vi "ExcelImport.vi"(8 "错误输入（无错误）":errorcluster, 10 "Sheets":enum16{"Sheet1", "Sheet2", "Sheet3", "Sheet4"}(ring), 11 "路径":path) -> (0 "错误输出":errorcluster, 1 "After First":string[][](array[string]), 2 "First Row":string[](array[string]), 3 "All":string[][](array[string]))   [LabVIEW 2020]
panel:
  out "x-y":u32
  in  "Excel._Worksheet":refnum<k7>
  in  "Excel._Application":refnum<k7>
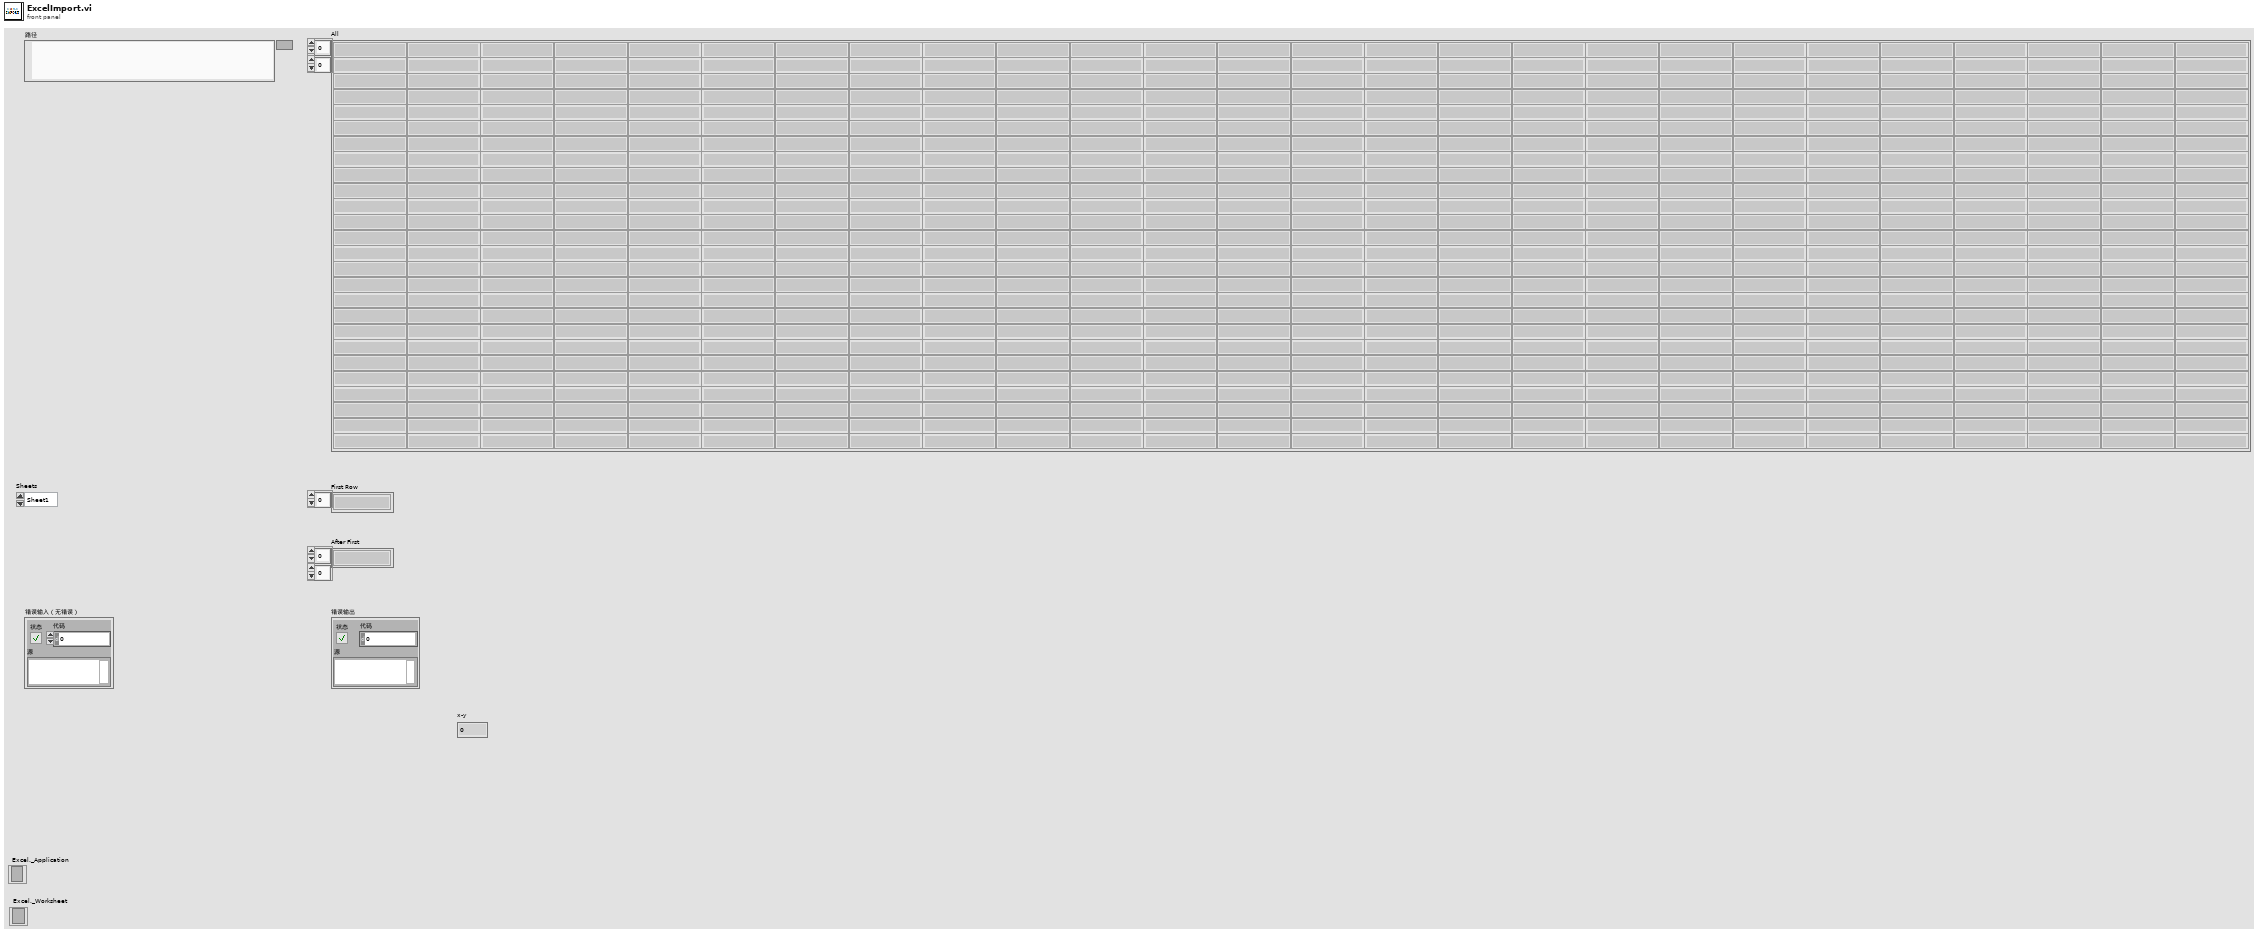
[diagram p1: front panel]
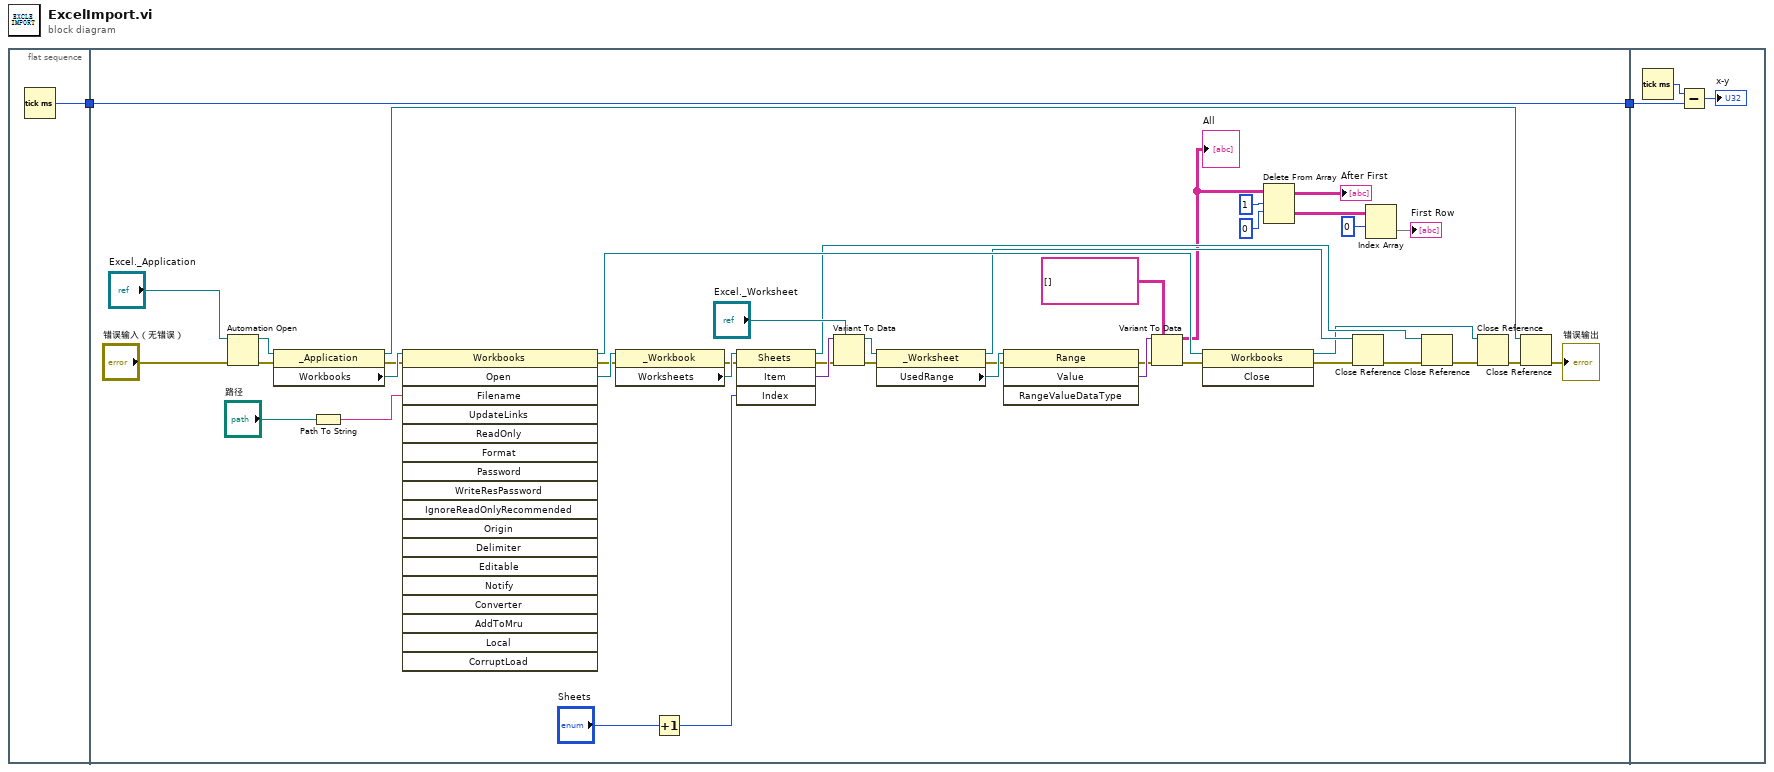
[diagram p0: block diagram]
diagram:
  n1 = flat-sequence {
    tunnel: [w3] -> w2
    tunnel: w2 -> [w10]
    tunnel: [w10] -> w1
    tunnel: w1 -> [w48]
    frame #0 {
      n2 = Tick Count (ms)() -> (millisecond timer value=w3:u32)
    }
    frame #1 {
      n3 = Automation Open(error in (no error)="错误输入（无错误）", Automation Refnum="Excel._Application") -> (Automation Refnum=w46:refnum<k7>, error out=w30:errorcluster)  [unwired: 2 in]
      n4 = property on="属性节点" class="_Application"(reference=w46, error in=w30) -> (reference out=w15:refnum<k7>, error out=w29:errorcluster, "Workbooks"=w44:refnum<k7>)
      n5 = Path To String(path="路径") -> (string=w42:string)
      n6 = invoke class="Workbooks" method="Open"(reference=w44, error in=w29, "Filename"=w42) -> (reference out=w32:refnum<k7>, error out=w28:errorcluster, "Open"=w41:refnum<k7>)  [unwired: 15 in, 15 out]
      n7 = property class="_Workbook"(reference=w41, error in=w28) -> (error out=w27:errorcluster, "Worksheets"=w40:refnum<k7>)  [unwired: 1 out]
      n8 = Increment(x="Sheets") -> (x+1=w11:enum16{"Sheet1", "Sheet2", "Sheet3", "Sheet4"})
      n9 = invoke class="Sheets" method="Item"(reference=w40, error in=w27, "Index"=w11) -> (reference out=w18:refnum<k7>, error out=w26:errorcluster, "Item"=w38:variant)  [unwired: 1 in, 1 out]
      n10 = Variant To Data(error in=w26, type="Excel._Worksheet", Variant=w38) -> (data=w37:refnum<k7>, error out=w25:errorcluster)
      n11 = property class="_Worksheet"(reference=w37, error in=w25) -> (reference out=w19:refnum<k7>, error out=w24:errorcluster, "UsedRange"=w36:refnum<k7>)
      n12 = invoke class="Range" method="Value"(reference=w36, error in=w24) -> (error out=w23:errorcluster, "Value"=w35:variant)  [unwired: 2 in, 2 out]
      n13 = Variant To Data(error in=w23, type=string[][] [], Variant=w35) -> (data=w8:string[][], error out=w31:errorcluster)
      "All" <- w8
      n14 = invoke class="Workbooks" method="Close"(reference=w32, error in=w31) -> (reference out=w17:refnum<k7>, error out=w22:errorcluster)  [unwired: 1 in, 1 out]
      n15 = Delete From Array(array=w8, length=1 ("长度"), index (row)=0 ("索引 (行)")) -> (deleted portion=w5:string[][], array with subset deleted=→"After First":string[][])  [unwired: 1 in]
      n16 = Close Reference(reference=w19, error in (no error)=w22) -> (error out=w21:errorcluster)
      n17 = Index Array(array=w5, index (row)=0 ("索引 (行)")) -> (element=→"First Row":string[])  [unwired: 1 in]
      n18 = Close Reference(reference=w18, error in (no error)=w21) -> (error out=w20:errorcluster)
      n19 = Close Reference(reference=w17, error in (no error)=w20) -> (error out=w16:errorcluster)
      n20 = Close Reference(reference=w15, error in (no error)=w16) -> (error out=→"错误输出":errorcluster)
    }
    frame #2 {
      n21 = Tick Count (ms)() -> (millisecond timer value=w49:u32)
      n22 = Subtract(x=w49, y=w48) -> (x-y=→"x-y":u32)
    }
  }
